vi "Sensor Data.vi"() -> ()   [LabVIEW 2016]
panel:
  out "Right Drive Encoder":dbl
  out "Left Drive Encoder":dbl
  out "Gear IR":bool
  out "Angle X":dbl
  out "Ball Conveyor Velocity":dbl
  out "Shooter Velocity":dbl
  out "Right Drive Velocity":dbl
  out "Left Drive Velocity":dbl
  out "IMU Heading":dbl
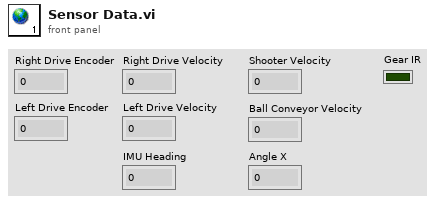
[diagram p1: front panel]
diagram:
